vi "Graph R and G vs Parameter.vi"(8 "indices":T1, 9 "AO Amp (V)":dbl[](array[numeric]), 10 "Y vs Parameter":cluster{"X-array":dbl[], "Y-array":dbl[]}[](array[cluster]), 11 "X vs Parameter":cluster{"X-array":dbl[], "Y-array":dbl[]}[](array[cluster])) -> (2 "G(Siemens) vs Parameter":cluster{"X-array":dbl[], dbl[]}[](array[cluster]), 3 "R(Ohms) vs Parameter":cluster{"X-array":dbl[], dbl[]}[](array[cluster]))   [LabVIEW 2019, in "Transport.lvclass"]
uses:
  Transport.lvclass
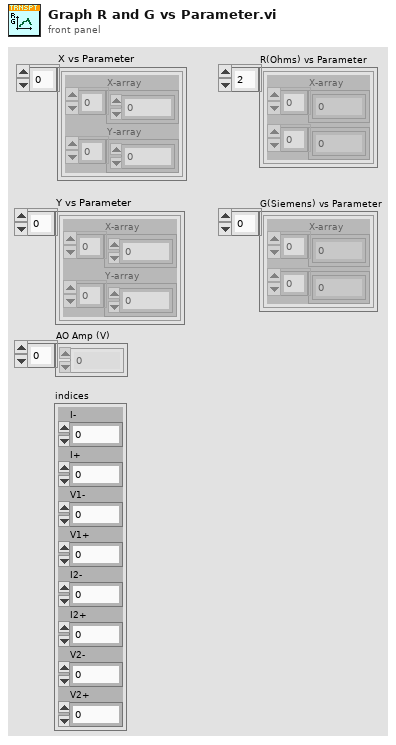
[diagram p1: front panel]
types:
  T1 = cluster{"I-":i32, "I+":i32, "V1-":i32, "V1+":i32, "I2-":i32, "I2+":i32, "V2-":i32, "V2+":i32}
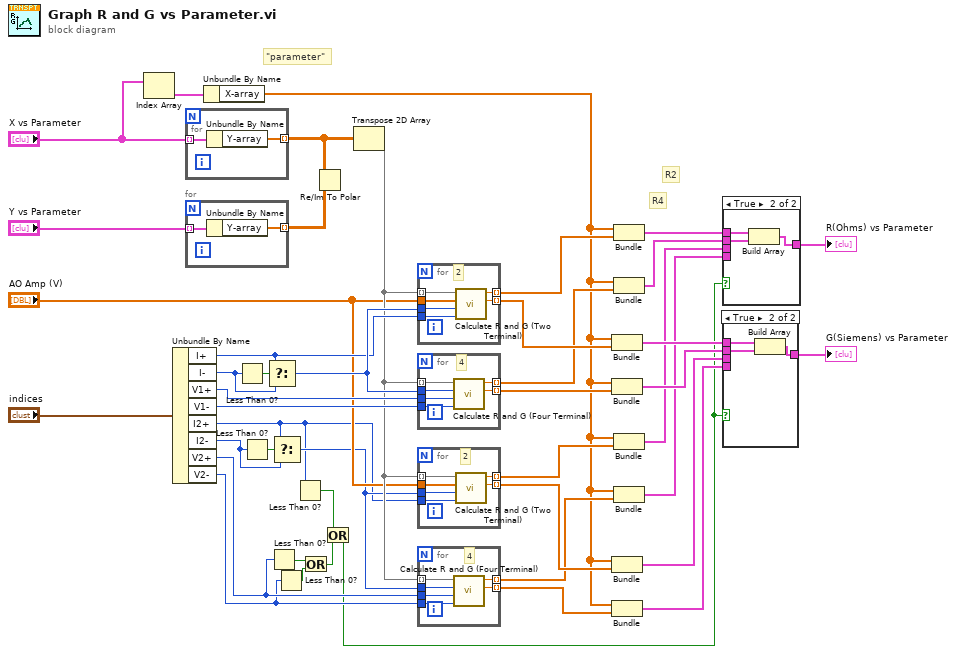
[diagram p0: block diagram]
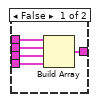
[diagram p2: hidden frame]
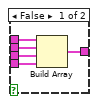
[diagram p3: hidden frame]
diagram:
  # "R4"
  # "R2"
  # "\"parameter\""
  n1 = Index Array(array="X vs Parameter") -> (element=w33:cluster{"X-array":dbl[], "Y-array":dbl[]})  [unwired: 1 in]
  n2 = Unbundle By Name("indices") -> ("I+"=w37:i32, "I-"=w38:i32, "V1+"=w35:i32, "V1-"=w34:i32, "I2+"=w9:i32, "I2-"=w20:i32, "V2+"=w8:i32, "V2-"=w7:i32)
  n3 = for {
    tunnel: "X vs Parameter" -> [w46] mode=indexing
    tunnel: [w45] -> w23 mode=indexing
    n4 = Unbundle By Name(w46) -> ("Y-array"=w45:dbl[])
  }
  n5 = for {
    tunnel: "Y vs Parameter" -> [w48] mode=indexing
    tunnel: [w47] -> w25 mode=indexing
    n6 = Unbundle By Name(w48) -> ("Y-array"=w47:dbl[])
  }
  n7 = Unbundle By Name(w33) -> ("X-array"=w4:dbl[])
  n8 = Less Than 0?(x=w38) -> (x < 0?=w36:bool)
  n9 = Less Than 0?(x=w20) -> (x < 0?=w21:bool)
  n10 = Select(t=w37, s=w36, f=w38) -> (s? t:f=w39:i32)
  n11 = Less Than 0?(x=w8) -> (x < 0?=w6:bool)
  n12 = Select(t=w9, s=w21, f=w20) -> (s? t:f=w18:i32)
  n13 = Less Than 0?(x=w7) -> (x < 0?=w5:bool)
  n14 = Less Than 0?(x=w9) -> (x < 0?=w3:bool)
  n15 = Or(x=w6, y=w5) -> (x .or. y?=w2:bool)
  n16 = Re/Im To Polar(2:w25, 3:w23) -> ()  [unwired: 2 out]
  n17 = Or(x=w3, y=w2) -> (x .or. y?=w1:bool)
  n18 = Transpose 2D Array(2D array=w23) -> (transposed array=w22:dbl[][])
  n19 = for {
    tunnel: w37 -> [w54]
    tunnel: w39 -> [w53]
    tunnel: w22 -> [w52] mode=indexing
    tunnel: [w51] -> w41 mode=indexing
    tunnel: [w50] -> w44 mode=indexing
    tunnel: "AO Amp (V)" -> [w49]
    # "2"
    n20 = call "Calculate R and G (Two Terminal).vi"("Vsource"=w54, "Current"=w53, "AO Amp (V)"=w49, "Lockin []"=w52) -> ("G_2T (Siemens)"=w50:dbl, "R_2T (Ohms)"=w51:dbl)  [unwired: 6 in]
  }
  n21 = for {
    tunnel: w34 -> [w60]
    tunnel: w35 -> [w59]
    tunnel: w39 -> [w58]
    tunnel: w22 -> [w57] mode=indexing
    tunnel: [w56] -> w43 mode=indexing
    tunnel: [w55] -> w42 mode=indexing
    # "4"
    n22 = call "Calculate R and G (Four Terminal).vi"("V-"=w60, "V+"=w59, "Current"=w58, "Lockin[ ]"=w57) -> ("G_4T (Siemens)"=w55:dbl, "R_4T (ohms)"=w56:dbl)  [unwired: 4 in, 2 out]
  }
  n23 = for {
    tunnel: w9 -> [w66]
    tunnel: w18 -> [w65]
    tunnel: w22 -> [w64] mode=indexing
    tunnel: [w63] -> w17 mode=indexing
    tunnel: [w62] -> w16 mode=indexing
    tunnel: "AO Amp (V)" -> [w61]
    # "2"
    n24 = call "Calculate R and G (Two Terminal).vi"("Vsource"=w66, "Current"=w65, "AO Amp (V)"=w61, "Lockin []"=w64) -> ("G_2T (Siemens)"=w62:dbl, "R_2T (Ohms)"=w63:dbl)  [unwired: 6 in]
  }
  n25 = for {
    tunnel: w7 -> [w72]
    tunnel: w8 -> [w71]
    tunnel: w18 -> [w70]
    tunnel: w22 -> [w69] mode=indexing
    tunnel: [w68] -> w15 mode=indexing
    tunnel: [w67] -> w14 mode=indexing
    # "4"
    n26 = call "Calculate R and G (Four Terminal).vi"("V-"=w72, "V+"=w71, "Current"=w70, "Lockin[ ]"=w69) -> ("G_4T (Siemens)"=w67:dbl, "R_4T (ohms)"=w68:dbl)  [unwired: 4 in, 2 out]
  }
  n27 = Bundle("X-array"=w4, w44) -> (w27:cluster{"X-array":dbl[], dbl[]})  [unwired: 1 in]
  n28 = Bundle("X-array"=w4, w42) -> (w29:cluster{"X-array":dbl[], dbl[]})  [unwired: 1 in]
  n29 = Bundle("X-array"=w4, w16) -> (w11:cluster{"X-array":dbl[], dbl[]})  [unwired: 1 in]
  n30 = Bundle("X-array"=w4, w14) -> (w10:cluster{"X-array":dbl[], dbl[]})  [unwired: 1 in]
  n31 = Bundle("X-array"=w4, w41) -> (w31:cluster{"X-array":dbl[], dbl[]})  [unwired: 1 in]
  n32 = Bundle("X-array"=w4, w43) -> (w30:cluster{"X-array":dbl[], dbl[]})  [unwired: 1 in]
  n33 = Bundle("X-array"=w4, w17) -> (w13:cluster{"X-array":dbl[], dbl[]})  [unwired: 1 in]
  n34 = Bundle("X-array"=w4, w15) -> (w12:cluster{"X-array":dbl[], dbl[]})  [unwired: 1 in]
  n35 = case shown="True" w1 {
    tunnel: [w77 w80] -> w32
    tunnel: w31 -> [w76 w79]
    tunnel: w30 -> [w75 w78]
    tunnel: w13 -> [w74 _]
    tunnel: w12 -> [w73 _]
    frame False {
      n36 = Build Array(w76, w75, w74, w73) -> (w77:cluster{"X-array":dbl[], dbl[]}[])
    }
    frame True {
      n37 = Build Array(w79, w78) -> (w80:cluster{"X-array":dbl[], dbl[]}[])
    }
  }
  "R(Ohms) vs Parameter" <- w32
  n38 = case shown="True" w1 {
    tunnel: w29 -> [w85 w88]
    tunnel: [w84 w87] -> w28
    tunnel: w27 -> [w83 w86]
    tunnel: w11 -> [w82 _]
    tunnel: w10 -> [w81 _]
    frame False {
      n39 = Build Array(w83, w85, w82, w81) -> (w84:cluster{"X-array":dbl[], dbl[]}[])
    }
    frame True {
      n40 = Build Array(w86, w88) -> (w87:cluster{"X-array":dbl[], dbl[]}[])
    }
  }
  "G(Siemens) vs Parameter" <- w28
